vi "Find Most Severe Subsystem Status.vi"(11 "Array":T1[](array[typedef])) -> (3 "Subystem Status":T1)   [LabVIEW 2014]
uses:
  Subsystem Status.ctl
  Subsystem Status Severity.ctl
  Subsystem Status Message.ctl
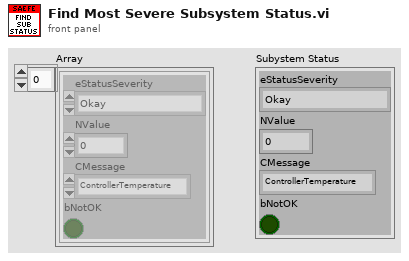
[diagram p1: front panel]
types:
  T1 = typedef "Subsystem Status.ctl" = cluster{"eStatusSeverity":T2, "NValue":sgl, "CMessage":T3, "bNotOK":bool}
  T2 = typedef "Subsystem Status Severity.ctl" = enum16{"Okay", "Short Warning", "Long Warning", "Return to Pits", "Error", "Danger"}
  T3 = typedef "Subsystem Status Message.ctl" = enum16{"ControllerTemperature", "MotorTemperature", "BatteryTemperature", "BatteryLowVoltage", "LVBattery", "sbRIOTemperature", "Precharge", "BSPD", "IMD", "RemoteReturnToPits", "EStopInterrupted", "NoCellComms", "MCOverSpeed", "MCOverCurrent", "MCOverVoltage", "MCInverterOverTemp", "MCDirectionCommand", "MCInverterTimeout", "MCDesatFault", "MCHWOverCurrent", "MCUnderVoltage", "MCCommandMessageLost", "MotorOverTemp", "MCModAOverTemp", "MCModBOverTemp", "MCModCOverTemp", "MCPCBOverTemp", "MCGateDrv1OverTemp", "MCDateDrv2OverTemp", "MCCurrentSensorFault", "MCResolverNotConnected", "ShutdownLatchTripped", "UnknownBMS", "RemoteEmergency"}
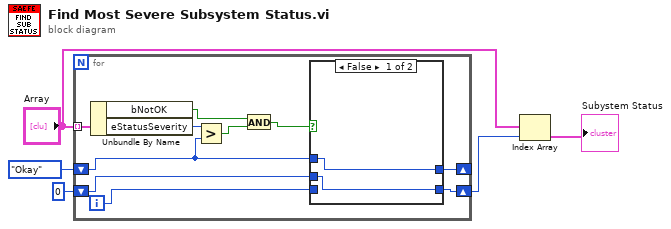
[diagram p0: block diagram]
diagram:
  n1 = for {
    tunnel: "Array" -> [w15] mode=indexing
    shift-right: [w10] -> _
    shift-left: Subsystem_Status_Severity."Okay" ("Status Severity") -> [w9]
    shift-right: [w12] -> w4
    shift-left: 0 -> [w11]
    i -> [w13]
    n2 = Unbundle By Name(w15) -> ("bNotOK"=w8:bool, "eStatusSeverity"=w14:T2)
    n3 = Greater?(x=w14, y=w9) -> (0:w7:bool)
    n4 = And(x=w8, y=w7) -> (x .and. y?=w6:bool)
    n5 = case shown="False" w6 {
      tunnel: w13 -> [_ w19]
      tunnel: [w17 w19] -> w12
      tunnel: w11 -> [w17 _]
      tunnel: w9 -> [w16 w18]
      tunnel: [w16 w18] -> w10
      frame False {
      }
      frame True {
      }
    }
  }
  n6 = Index Array(array="Array", index=w4) -> (element=→"Subystem Status":T1)
